vi "Make DLL Param(Read Req).vi"   [LabVIEW 2014, in "Keyence LJ-V7000.lvlib"]
uses:
  Keyence LJ-V7000.lvlib
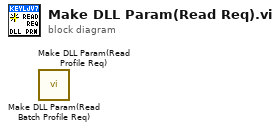
[diagram p0: block diagram]
diagram:
  n1 = call "Make DLL Param(Read Batch Profile Req).vi"() -> ()  [unwired: 1 in, 1 out]
  n2 = call "Make DLL Param(Read Profile Req).vi"() -> ()  [unwired: 1 in, 1 out]
